vi "get_and_correct_crossings.vi"(8 "dt":dbl, 9 "peak times":dbl[](array[numeric]), 10 "signal index":dbl[](array[numeric]), 11 "singal":dbl[](array[numeric])) -> (1 "p->n crossing?":bool[](array[boolean]), 2 "n->p crossing?":bool[](array[boolean]), 3 "crossings":dbl[](array[numeric]), 4 "p->n indexes":i32[](array[numeric]), 6 "n->p indexes":i32[](array[numeric]))   [LabVIEW 2019]
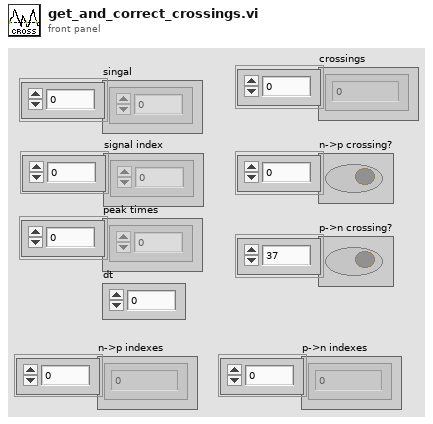
[diagram p1: front panel]
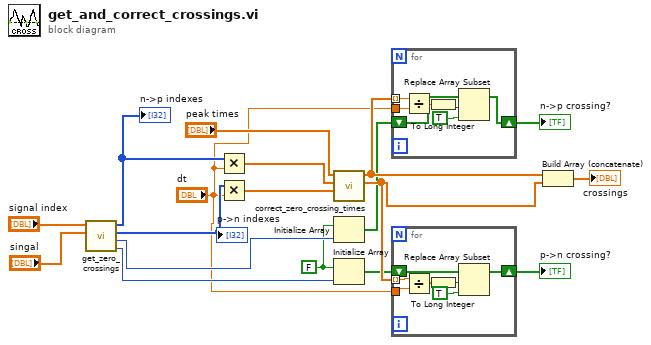
[diagram p0: block diagram]
diagram:
  w2 = FALSE
  n1 = call "get_zero_crossings.vi"("signal"="singal", "index"="signal index") -> ("size of p->n array"=w18:i32, "size of n->p array"=w17:i32, "p->n indexes"=w16:i32[], "n->p indexes"=w15:i32[])  [unwired: 5 in]
  "p->n indexes" <- w16
  "n->p indexes" <- w15
  n2 = Multiply(x=w15, y="dt") -> (x*y=w12:dbl[])
  n3 = Multiply(x=w16, y="dt") -> (x*y=w9:dbl[])
  n4 = call "correct_zero_crossing_times.vi"("p->n idõk"=w9, "n->p idõk"=w12, "csúcs idõk"="peak times") -> ("korrigált p->n idõk"=w8:dbl[], "korrigált n->p idõk"=w7:dbl[])  [unwired: 7 in]
  n5 = Initialize Array(w2, w17) -> (w3:bool[])
  n6 = Initialize Array(w2, w18) -> (w5:bool[])
  n7 = for {
    tunnel: w7 -> [w22] mode=indexing
    shift-right: [w24] -> w4
    shift-left: w3 -> [w25]
    tunnel: "dt" -> [w21]
    n8 = Divide(x=w22, y=w21) -> (x/y=w20:dbl)
    n9 = To Long Integer(number=w20) -> (32bit integer=w19:i32)
    n10 = Replace Array Subset(array=w25, new element=TRUE, index=w19) -> (w24:bool[])
  }
  "n->p crossing?" <- w4
  n11 = for {
    tunnel: w8 -> [w27] mode=indexing
    shift-right: [w31] -> w6
    shift-left: w5 -> [w32]
    tunnel: "dt" -> [w26]
    n12 = Divide(x=w27, y=w26) -> (x/y=w28:dbl)
    n13 = To Long Integer(number=w28) -> (32bit integer=w29:i32)
    n14 = Replace Array Subset(array=w32, new element=TRUE, index=w29) -> (w31:bool[])
  }
  "p->n crossing?" <- w6
  n15 = Build Array (concatenate)(w7, w8) -> (→"crossings":dbl[])
